vi "R3_Control-REVISED.vi"() -> ()   [LabVIEW 2016]
uses:
  R3 Reactor Status v1.ctl
  R3 PR pH Manual Control.ctl
  R3 Pump Manual Control.ctl
  R3Variables.lvlib
panel:
  in  "R3 PR pH Manual Control":T1
  out "pH and DO":T2(graph)
  in  "pH AR  Manual Control":bool
  out "AR pH Intercept":dbl
  out "AR pH slope":dbl
  in  "AR pH Calibrate":bool
  in  "Reactor 3 AR pH Manual Control":T3
  in  "AR pH Control":T4={" pH Set Point"=7.5, " pH Tolerance"=0.1, "Reaction Time (s)"=15.0, "Pump On Time (s)"=3.0}
  in  "SBR Timing":T5={"AR feeding"=0.0, "AR Decant"=0.0, "Anoxic feeding (min)"=40.0, "Anaerobic Time (min)"=53.0, "Anaerobic feeding (min)"=5.0, "Anoxic Time (min)"=60.0, "Aerobic Time (min) "=60.0, "Settle (min)"=20.0, "Decant (min)"=2.0}
  in  "R3 Pumps Manual Control":T6
  out "R3 Reactor Status":T7 {"DO (mg/L)" format="%#_3g"; "pH 1" format="%#_3g"}
  out "Elapsed Time":dbl
  out "DO Intercept":dbl
  out "DO Slope":dbl
  out "PR pH Intercept":dbl
  out "PR pH Slope":dbl
  in  "PR pH Control":T4={" pH Set Point"=7.5, " pH Tolerance"=0.1, "Reaction Time (s)"=15.0, "Pump On Time (s)"=3.0}
  in  "Pumps Manual Control":bool
  in  "pH PR Manual Control":bool
  in  "DO Calibrate":bool
  in  "PR pH Calibrate":bool
  # "On: Manual Mode\nOff: SBR Mode"
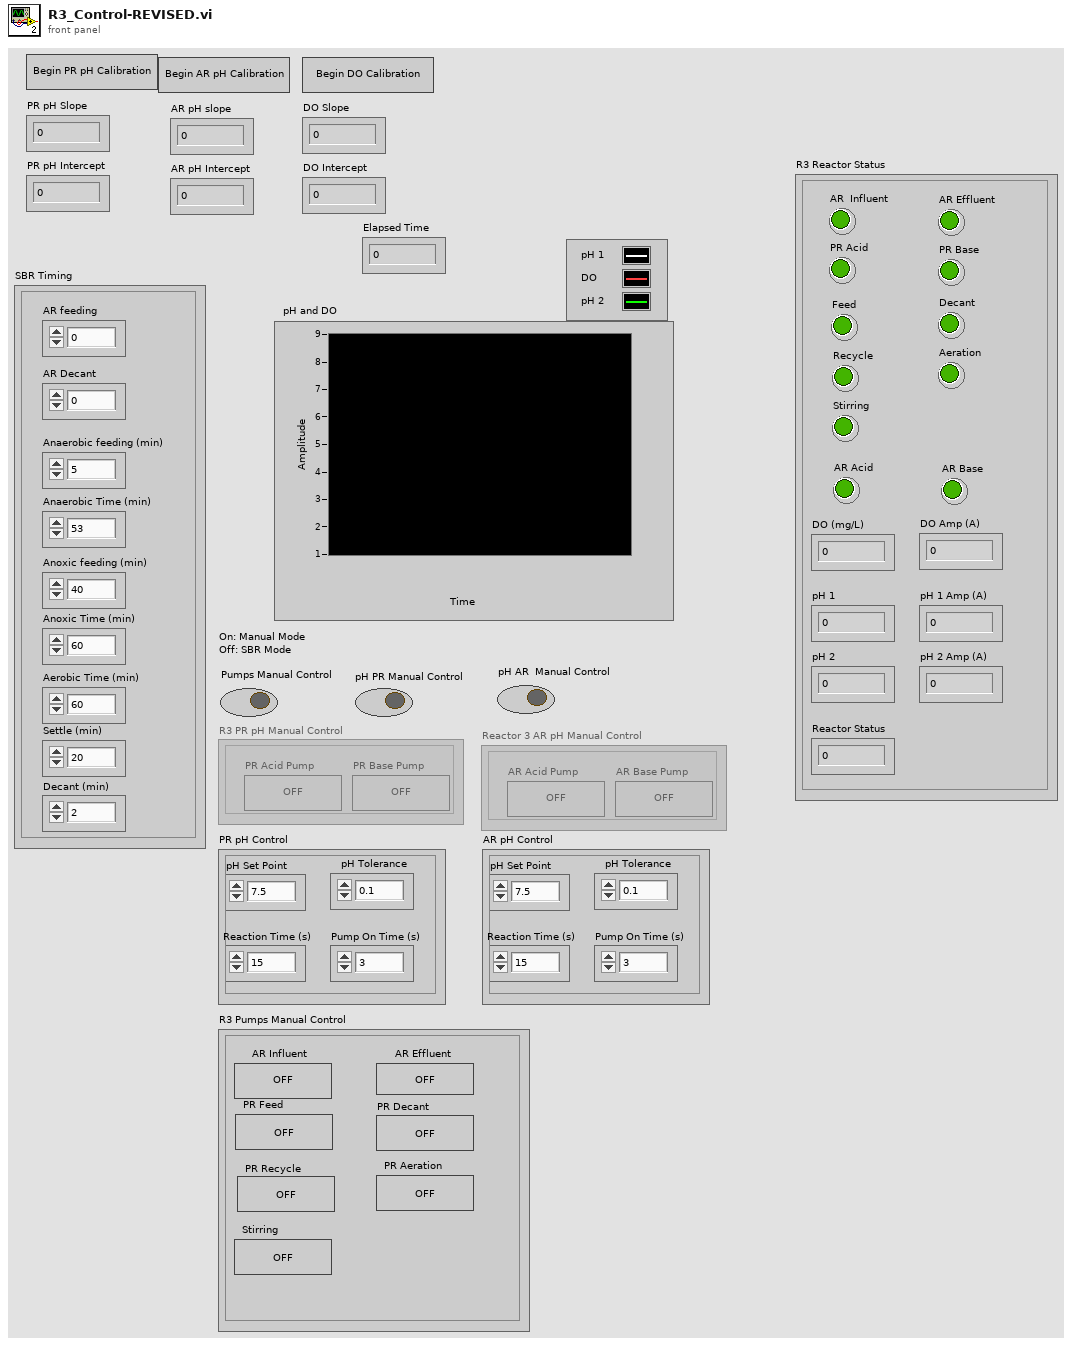
[diagram p1: front panel]
types:
  T1 = typedef "R3Variables.lvlib/R3 PR pH Manual Control.ctl" = cluster{"PR Acid Pump":bool, "PR Base Pump":bool}
  T2 = cluster{"pH 1 Amp (A)":dbl, "DO (mg/L)":dbl, "pH 2 Amp (A)":dbl}
  T3 = cluster{"AR Acid Pump":bool, "AR Base Pump":bool}
  T4 = cluster{" pH Set Point":dbl, " pH Tolerance":dbl, "Reaction Time (s)":dbl, "Pump On Time (s)":dbl}
  T5 = cluster{"AR feeding":dbl, "AR Decant":dbl, "Anoxic feeding (min)":dbl, "Anaerobic Time (min)":dbl, "Anaerobic feeding (min)":dbl, "Anoxic Time (min)":dbl, "Aerobic Time (min) ":dbl, "Settle (min)":dbl, "Decant (min)":dbl}
  T6 = cluster{"AR Influent":bool, "AR Effluent":bool, "PR Feed":bool, "PR Decant":bool, "PR Recycle":bool, "PR Aeration":bool, "Stirring":bool}
  T7 = typedef "R3Variables.lvlib/R3 Reactor Status v1.ctl" = cluster{"AR  Influent":bool, "AR Effluent":bool, "PR Acid":bool, "PR Base":bool, "Feed":bool, "Aeration":bool, "Decant":bool, "pH 1":dbl, "DO (mg/L)":dbl, "pH 1 Amp (A)":dbl, "DO Amp (A)":dbl, "Recycle":bool, "Stirring":bool, "Reactor Status":dbl, "AR Acid":bool, "AR Base":bool, "pH 2":dbl, "pH 2 Amp (A)":dbl}
  T8 = cluster{"pH 1 Amp (A)":dbl, "DO (mg/L)":dbl, "pH 2 Amp (A)":dbl}[]
  T9 = enum8{"Enabled", "Disabled", "Disabled and Grayed Out"}
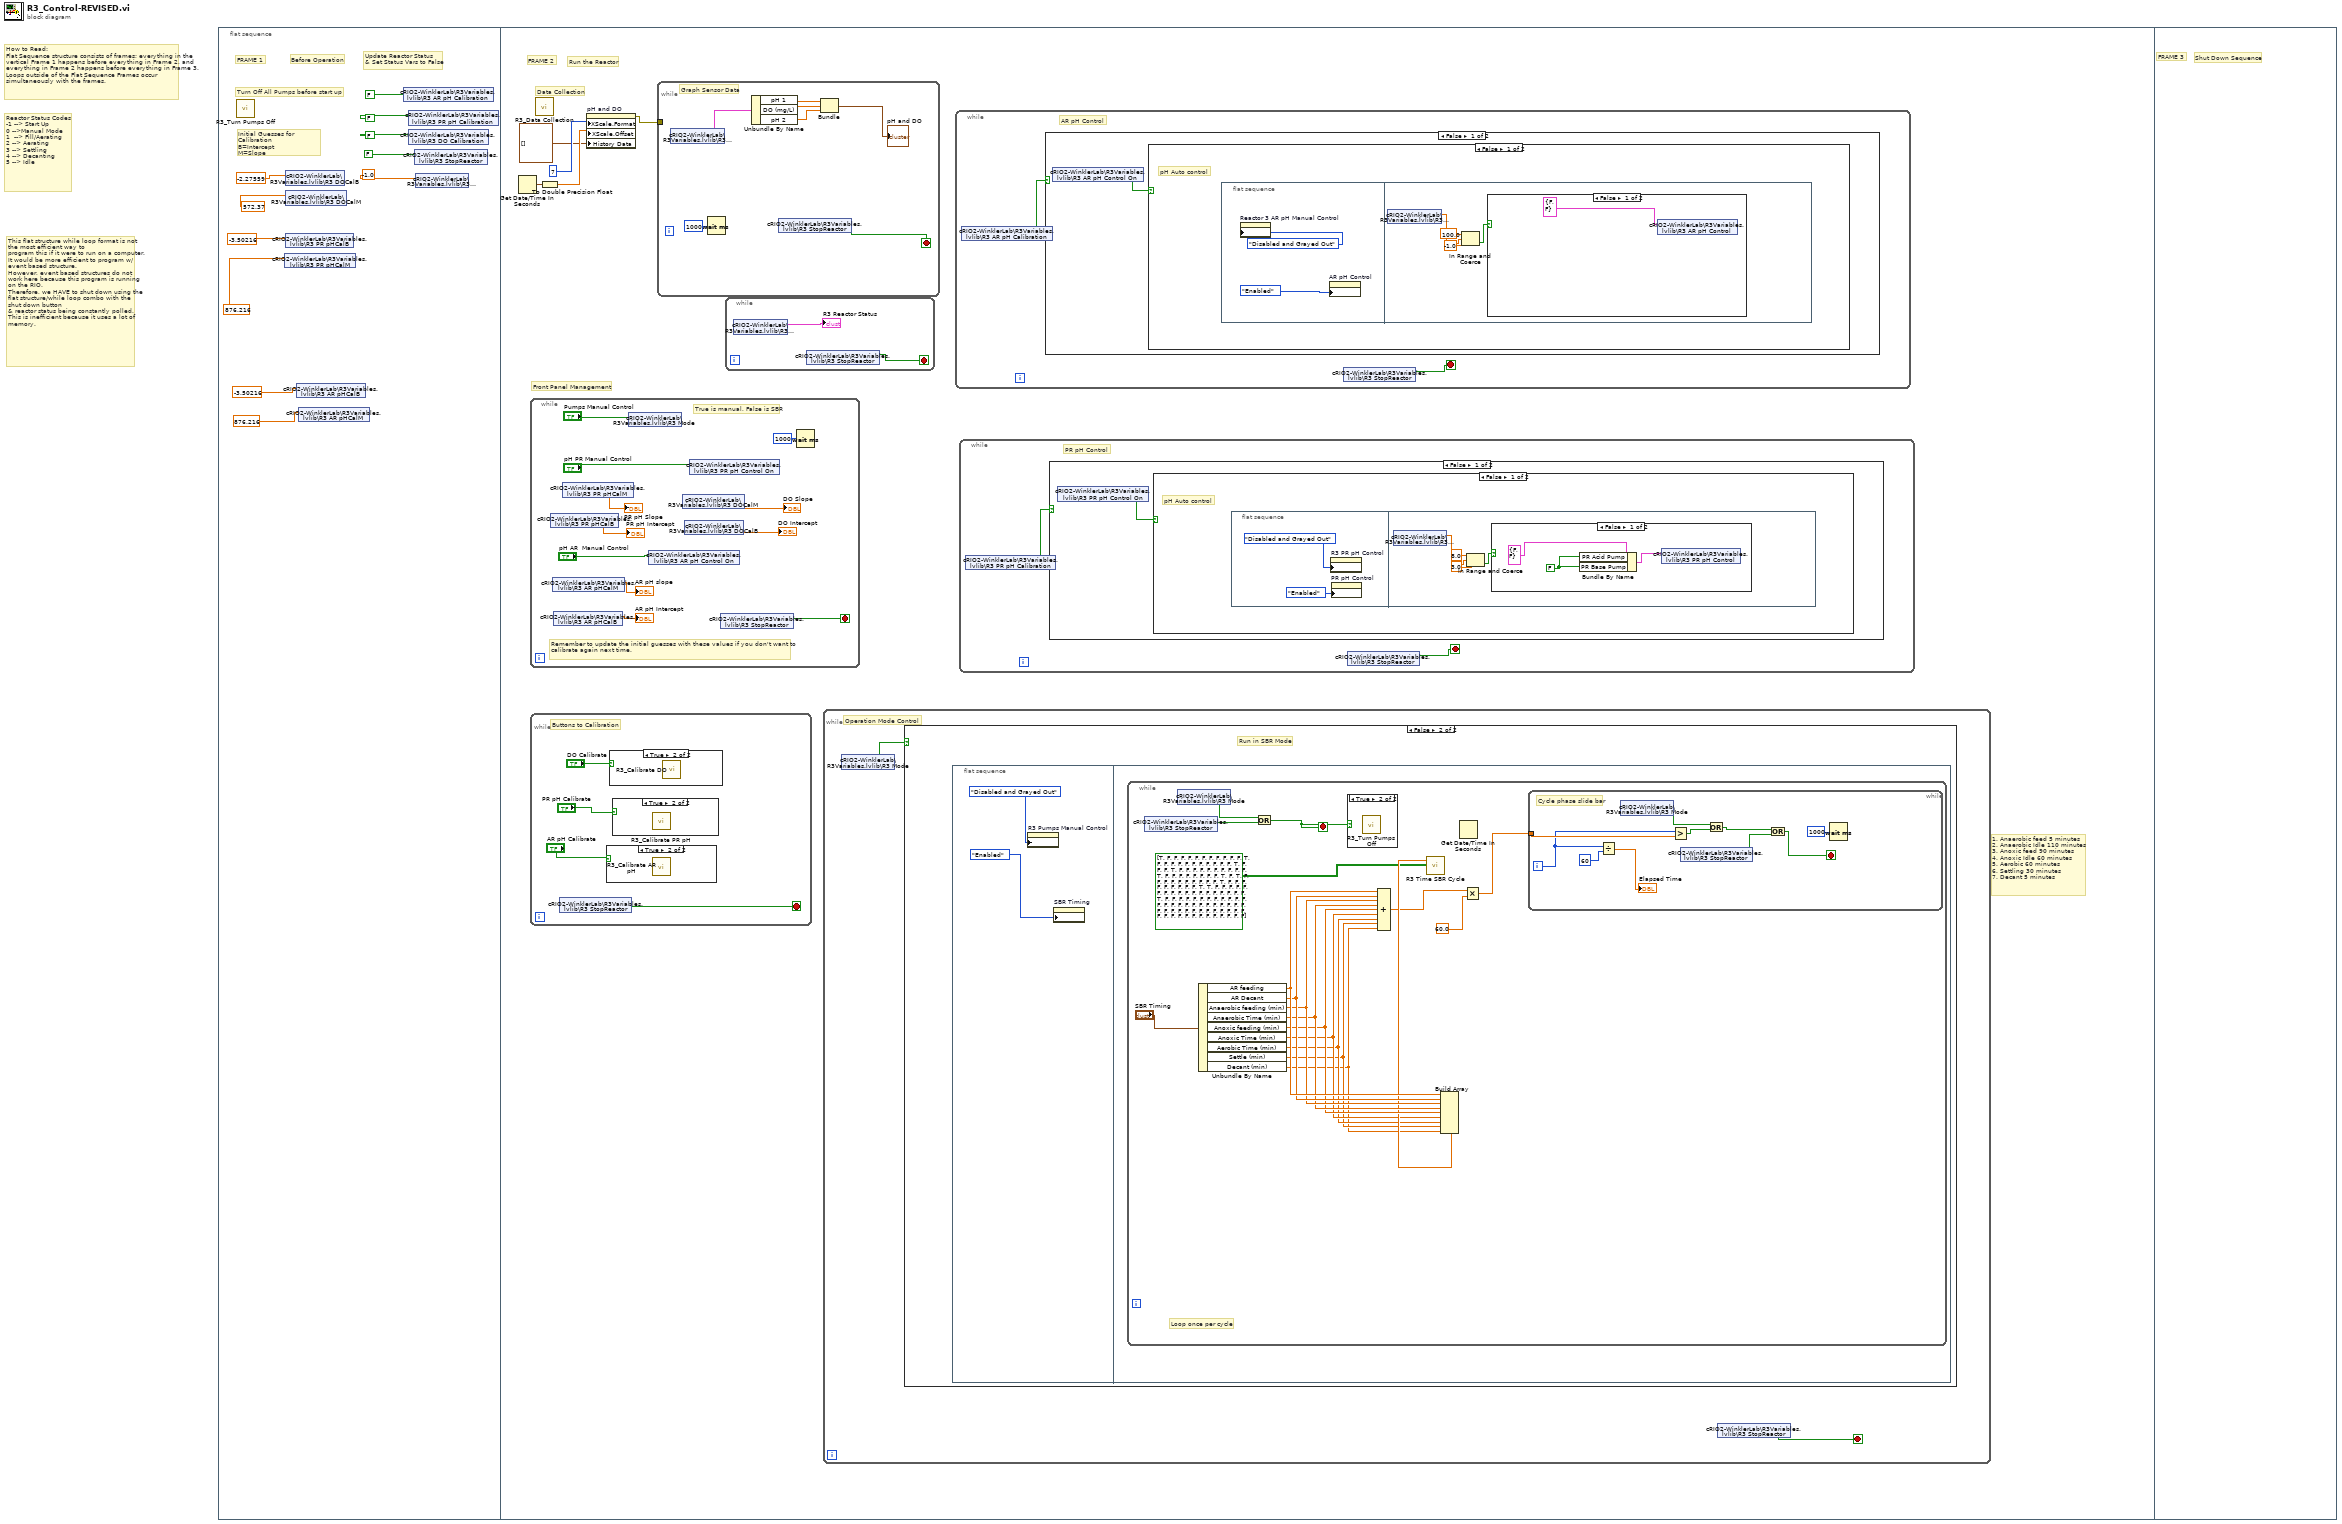
[diagram p0: block diagram]
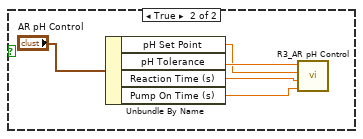
[diagram p2: hidden frame]
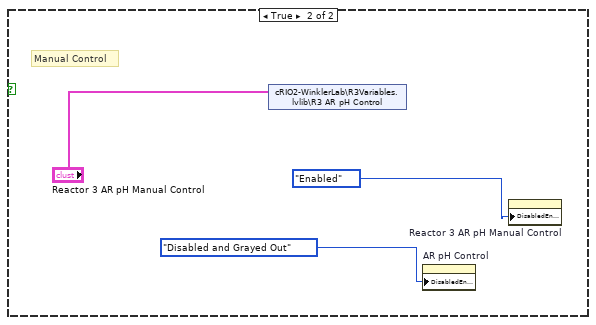
[diagram p3: hidden frame]
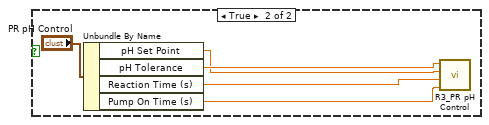
[diagram p8: hidden frame]
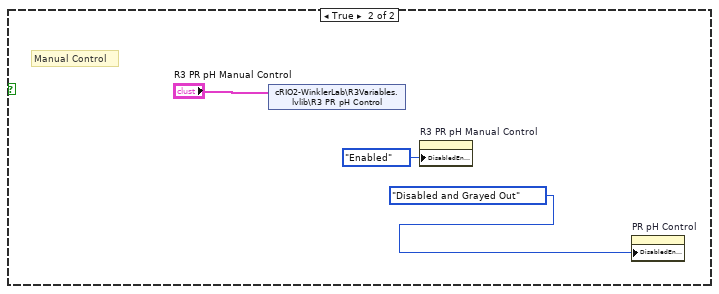
[diagram p9: hidden frame]
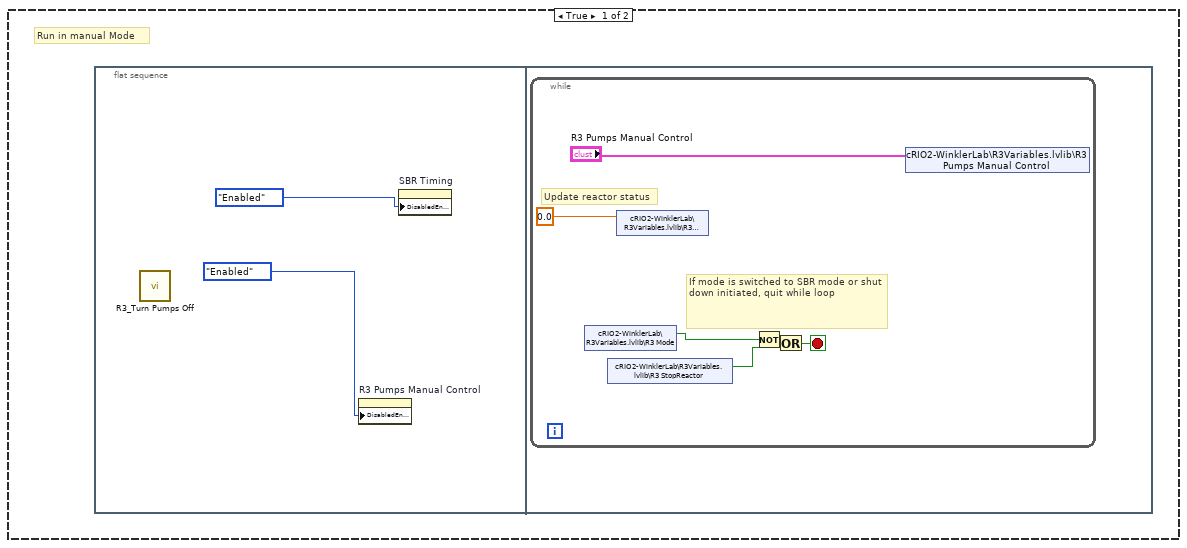
[diagram p11: hidden frame]
diagram:
  # "Reactor Status Codes\n-1 --> Start Up\n0 -->Manual Mode\n1  --> Fill/Aerating\n2 --> Aerating\n3 --> Settling\n4 --> Decanting\n5 --> Idle"
  # "How to Read:\nFlat Sequence structure consists of frames; everything in the vertical Frame 1 happens before everything in Frame 2, and everything in Frame 2 happens before everything in Frame 3.\nLoops outside of the Flat Sequence Frames occur simultaneously with the frames."
  # "This flat structure while loop format is not the most efficient way to \nprogram this if it were to run on a computer.\nIt would be more efficient to program w/ event based structure.\nHowever, event based structures do not work here because this program is running on the RIO.\nTherefore, we HAVE to shut down using the flat structure/while loop combo with the shut down button \n& reactor status being constantly polled.\nThis is inefficient because it uses a lot of memory."
  n1 = flat-sequence {
    frame #0 {
      # "Initial Guesses for Calibration\nB=Intercept\nM=Slope"
      # "Update Reactor Status \n& Set Status Vars to False"
      # "Turn Off All Pumps before start up"
      # "FRAME 1"
      # "Before Operation"
      n2 = call "R3_Turn Pumps Off.vi"() -> ()  [unwired: 12 in]
      n3 = shared-variable "cRIO2-WinklerLab\\R3Variables.lvlib\\R3 PR pHCalM"(876.216 ("R1pHCalM")) -> ()  [unwired: 1 in, 1 out]
      n4 = shared-variable "cRIO2-WinklerLab\\R3Variables.lvlib\\R3 DOCalB"(-2.27559 ("R1DOxCalB")) -> ()  [unwired: 1 in, 1 out]
      n5 = shared-variable "cRIO2-WinklerLab\\R3Variables.lvlib\\R3 DOCalM"(572.37 ("R1DOxCalM")) -> ()  [unwired: 1 in, 1 out]
      n6 = shared-variable "cRIO2-WinklerLab\\R3Variables.lvlib\\R3 PR pHCalB"(-3.50216 ("R1pHCalB")) -> ()  [unwired: 1 in, 1 out]
      n7 = shared-variable "cRIO2-WinklerLab\\R3Variables.lvlib\\R3 AR pHCalB"(-3.50216 ("pH Amperage")) -> ()  [unwired: 1 in, 1 out]
      n8 = shared-variable "cRIO2-WinklerLab\\R3Variables.lvlib\\R3 AR pHCalM"(876.216 ("Buffer Solution pH")) -> ()  [unwired: 1 in, 1 out]
      n9 = shared-variable "cRIO2-WinklerLab\\R3Variables.lvlib\\R3 AR pH Calibration"(FALSE ("Begin Calibration")) -> ()  [unwired: 1 in, 1 out]
      n10 = shared-variable "cRIO2-WinklerLab\\R3Variables.lvlib\\R3 PR pH Calibration"(FALSE ("pH Calibration")) -> ()  [unwired: 1 in, 1 out]
      n11 = shared-variable "cRIO2-WinklerLab\\R3Variables.lvlib\\R3 DO Calibration"(FALSE ("DO Calibration")) -> ()  [unwired: 1 in, 1 out]
      n12 = shared-variable "cRIO2-WinklerLab\\R3Variables.lvlib\\R3 StopReactor"(FALSE ("R1Stop Reactor")) -> ()  [unwired: 1 in, 1 out]
      n13 = shared-variable "cRIO2-WinklerLab\\R3Variables.lvlib\\R3 Phase"(-1.0) -> ()  [unwired: 1 in, 1 out]
    }
    frame #1 {
      # "1. Anaerobic feed 5 minutes\n2. Anaerobic Idle 110 minutes \n3. Anoxic feed 90 minutes\n4. Anoxic Idle 60 minutes\n5. Aerobic 60 minutes\n6. Settling 30 minutes\n7. Decant 5 minutes"
      # "Front Panel Management"
      # "Data Collection"
      # "FRAME 2"
      # "Run the Reactor"
      n14 = Get Date/Time In Seconds() -> (seconds since 1Jan1904=w16:timestamp)
      n15 = while {
        stop <- w75 stop-if-true
        # "Remember to update the initial guesses with these values if you don't want to calibrate again next time."
        # "True is manual, False is SBR"
        n16 = shared-variable "cRIO2-WinklerLab\\R3Variables.lvlib\\R3 PR pHCalB"() -> (→"PR pH Intercept":dbl)  [unwired: 1 in, 1 out]
        n17 = shared-variable "cRIO2-WinklerLab\\R3Variables.lvlib\\R3 AR pHCalM"() -> (→"AR pH slope":dbl)  [unwired: 1 in, 1 out]
        n18 = shared-variable "cRIO2-WinklerLab\\R3Variables.lvlib\\R3 AR pHCalB"() -> (→"AR pH Intercept":dbl)  [unwired: 1 in, 1 out]
        n19 = shared-variable "cRIO2-WinklerLab\\R3Variables.lvlib\\R3 PR pHCalM"() -> (→"PR pH Slope":dbl)  [unwired: 1 in, 1 out]
        n20 = shared-variable "cRIO2-WinklerLab\\R3Variables.lvlib\\R3 Mode"("Pumps Manual Control") -> ()  [unwired: 1 in, 1 out]
        n21 = shared-variable "cRIO2-WinklerLab\\R3Variables.lvlib\\R3 AR pH Control On"("pH AR  Manual Control") -> ()  [unwired: 1 in, 1 out]
        n22 = shared-variable "cRIO2-WinklerLab\\R3Variables.lvlib\\R3 DOCalM"() -> (→"DO Slope":dbl)  [unwired: 1 in, 1 out]
        n23 = shared-variable "cRIO2-WinklerLab\\R3Variables.lvlib\\R3 DOCalB"() -> (→"DO Intercept":dbl)  [unwired: 1 in, 1 out]
        n24 = shared-variable "cRIO2-WinklerLab\\R3Variables.lvlib\\R3 PR pH Control On"("pH PR Manual Control") -> ()  [unwired: 1 in, 1 out]
        n25 = shared-variable "cRIO2-WinklerLab\\R3Variables.lvlib\\R3 StopReactor"() -> (w75:bool)  [unwired: 1 in, 1 out]
        n26 = Wait (ms)(milliseconds to wait=u32 1000) -> ()  [unwired: 1 out]
      }
      n27 = while {
        stop <- w45 stop-if-true
        # "Buttons to Calibration"
        n28 = shared-variable "cRIO2-WinklerLab\\R3Variables.lvlib\\R3 StopReactor"() -> (w45:bool)  [unwired: 1 in, 1 out]
        n29 = case shown="True" "AR pH Calibrate" {
          frame False {
          }
          frame True {
            n30 = call "R3_Calibrate AR pH.vi"() -> ()  [unwired: 12 in]
          }
        }
        n31 = case shown="True" "DO Calibrate" {
          frame False {
          }
          frame True {
            n32 = call "R3_Calibrate DO.vi"() -> ()  [unwired: 12 in]
          }
        }
        n33 = case shown="True" "PR pH Calibrate" {
          frame False {
          }
          frame True {
            n34 = call "R3_Calibrate PR pH.vi"() -> ()  [unwired: 12 in]
          }
        }
      }
      n35 = call "R3_Data Collection.vi"() -> ()  [unwired: 12 in]
      n36 = To Double Precision Float(number=w16) -> (double precision float=w14:dbl)
      n37 = property on="pH and DO" class="WFChart (strict)"("XScale.Format"=u8 7 ("X Scale.Display Format:Format"), "XScale.Offset"=w14, "History Data"=T8 []) -> (error out=w13:errorcluster)  [unwired: 2 in, 1 out]
      n38 = while {
        tunnel: w13 -> [_]
        stop <- w41 stop-if-true
        # "Graph Sensor Data"
        n39 = shared-variable "cRIO2-WinklerLab\\R3Variables.lvlib\\R3 Status"() -> (w39:T7)  [unwired: 1 in, 1 out]
        n40 = Wait (ms)(milliseconds to wait=u32 1000) -> ()  [unwired: 1 out]
        n41 = Unbundle By Name(w39) -> ("pH 1"=w42:dbl, "DO (mg/L)"=w43:dbl, "pH 2"=w37:dbl)
        n42 = shared-variable "cRIO2-WinklerLab\\R3Variables.lvlib\\R3 StopReactor"() -> (w41:bool)  [unwired: 1 in, 1 out]
        n43 = Bundle("pH 1"=w42, "DO (mg/L)"=w43, "pH 2"=w37) -> (→"pH and DO":cluster{"pH 1":dbl, "DO (mg/L)":dbl, "pH 2":dbl})  [unwired: 1 in]
      }
      n44 = while {
        stop <- w36 stop-if-true
        n45 = shared-variable "cRIO2-WinklerLab\\R3Variables.lvlib\\R3 Status"() -> (→"R3 Reactor Status":T7)  [unwired: 1 in, 1 out]
        n46 = shared-variable "cRIO2-WinklerLab\\R3Variables.lvlib\\R3 StopReactor"() -> (w36:bool)  [unwired: 1 in, 1 out]
      }
      n47 = while {
        stop <- w80 stop-if-true
        # "Operation Mode Control"
        n48 = shared-variable "cRIO2-WinklerLab\\R3Variables.lvlib\\R3 Mode"() -> (w79:bool)  [unwired: 1 in, 1 out]
        n49 = case shown="False" w79 {
          frame True {
            # "Run in manual Mode"
            n50 = flat-sequence {
              frame #0 {
                n51 = call "R3_Turn Pumps Off.vi"() -> ()  [unwired: 12 in]
                n52 = property on="R3 Pumps Manual Control" class="Clust (strict)"("DisabledEnum"=T9."Enabled" ("Disabled")) -> ()  [unwired: 2 in, 2 out]
                n53 = property on="SBR Timing" class="Clust (strict)"("DisabledEnum"=T9."Enabled" ("Disabled")) -> ()  [unwired: 2 in, 2 out]
              }
              frame #1 {
                n54 = while {
                  stop <- w87 stop-if-true
                  # "If mode is switched to SBR mode or shut \ndown initiated, quit while loop"
                  # "Update reactor status"
                  n55 = shared-variable "cRIO2-WinklerLab\\R3Variables.lvlib\\R3 Mode"() -> (w85:bool)  [unwired: 1 in, 1 out]
                  n56 = shared-variable "cRIO2-WinklerLab\\R3Variables.lvlib\\R3 StopReactor"() -> (w84:bool)  [unwired: 1 in, 1 out]
                  n57 = shared-variable "cRIO2-WinklerLab\\R3Variables.lvlib\\R3 Phase"(0.0 ("Reactor Status")) -> ()  [unwired: 1 in, 1 out]
                  n58 = Not(x=w85) -> (.not. x?=w88:bool)
                  n59 = Or(x=w88, y=w84) -> (x .or. y?=w87:bool)
                  n60 = shared-variable "cRIO2-WinklerLab\\R3Variables.lvlib\\R3 Pumps Manual Control"("R3 Pumps Manual Control") -> ()  [unwired: 1 in, 1 out]
                }
              }
            }
          }
          frame False {
            # "Run in SBR Mode"
            n61 = flat-sequence {
              frame #0 {
                n62 = property on="R3 Pumps Manual Control" class="Clust (strict)"("DisabledEnum"=T9."Disabled and Grayed Out" ("Disabled")) -> ()  [unwired: 2 in, 2 out]
                n63 = property on="SBR Timing" class="Clust (strict)"("DisabledEnum"=T9."Enabled" ("Disabled")) -> ()  [unwired: 2 in, 2 out]
              }
              frame #1 {
                n64 = while {
                  stop <- w108 stop-if-true
                  # "Loop once per cycle"
                  n65 = shared-variable "cRIO2-WinklerLab\\R3Variables.lvlib\\R3 StopReactor"() -> (w106:bool)  [unwired: 1 in, 1 out]
                  n66 = shared-variable "cRIO2-WinklerLab\\R3Variables.lvlib\\R3 Mode"() -> (w107:bool)  [unwired: 1 in, 1 out]
                  n67 = Unbundle By Name("SBR Timing") -> ("AR feeding"=w105:dbl, "AR Decant"=w104:dbl, "Anaerobic feeding (min)"=w103:dbl, "Anaerobic Time (min)"=w102:dbl, "Anoxic feeding (min)"=w101:dbl, "Anoxic Time (min)"=w95:dbl, "Aerobic Time (min)"=w94:dbl, "Settle (min)"=w93:dbl, "Decant (min)"=w92:dbl)
                  n68 = Or(x=w107, y=w106) -> (x .or. y?=w108:bool)
                  n69 = case shown="True" w108 {
                    frame False {
                    }
                    frame True {
                      n70 = call "R3_Turn Pumps Off.vi"() -> ()  [unwired: 12 in]
                    }
                  }
                  n71 = Compound Arithmetic op=ADD(w105, w104, w103, w102, w101, w95, w94, w93, w92) -> (w96:dbl)
                  n72 = Build Array(w105, w104, w103, w102, w101, w95, w94, w93, w92) -> (w100:dbl[])
                  n73 = call "R3 Time SBR Cycle.vi"("Pump Status Array"=bool[][] [[TRUE, FALSE, FALSE, FALSE, FALSE, FALSE, FALSE, FALSE, FALSE, FALSE, FALSE], [FALSE, TRUE, FALSE, FALSE, FALSE, FALSE, FALSE, FALSE, FALSE, FALSE, FALSE], [FALSE, FALSE, TRUE, FALSE, FALSE, FALSE, TRUE, FALSE, FALSE, FALSE, FALSE], [FALSE, FALSE, FALSE, FALSE, FALSE, FALSE, TRUE, FALSE, FALSE, FALSE, FALSE], [FALSE, FALSE, FALSE, FALSE, TRUE, FALSE, TRUE, FALSE, FALSE, FALSE, FALSE], [FALSE, FALSE, FALSE, FALSE, FALSE, FALSE, TRUE, FALSE, FALSE, FALSE, FALSE], [FALSE, FALSE, FALSE, FALSE, FALSE, TRUE, TRUE, FALSE, FALSE, FALSE, FALSE], [FALSE, FALSE, FALSE, FALSE, FALSE, FALSE, FALSE, FALSE, FALSE, FALSE, FALSE], [FALSE, FALSE, FALSE, TRUE, FALSE, FALSE, FALSE, FALSE, FALSE, FALSE, FALSE], [FALSE, FALSE, FALSE, FALSE, FALSE, FALSE, FALSE, FALSE, FALSE, FALSE, FALSE], [FALSE, FALSE, FALSE, FALSE, FALSE, FALSE, FALSE, FALSE, FALSE, FALSE, FALSE], [FALSE, FALSE, FALSE, FALSE, FALSE, FALSE, FALSE, FALSE, FALSE, FALSE, FALSE], [FALSE, FALSE, FALSE, FALSE, FALSE, FALSE, FALSE, FALSE, FALSE, FALSE, FALSE]], "Timing Array"=w100) -> ()  [unwired: 10 in]
                  n74 = Get Date/Time In Seconds() -> ()  [unwired: 1 out]
                  n75 = Multiply(x=w96, y=60.0) -> (x*y=w97:dbl)
                  n76 = while {
                    tunnel: w97 -> [w117]
                    i -> [w111]
                    stop <- w112 stop-if-true
                    # "Cycle phase slide bar"
                    n77 = Divide(x=w111, y=60) -> (x/y=→"Elapsed Time":dbl)
                    n78 = shared-variable "cRIO2-WinklerLab\\R3Variables.lvlib\\R3 Mode"() -> (w114:bool)  [unwired: 1 in, 1 out]
                    n79 = Greater?(x=w111, y=w117) -> (0:w115:bool)
                    n80 = shared-variable "cRIO2-WinklerLab\\R3Variables.lvlib\\R3 StopReactor"() -> (w109:bool)  [unwired: 1 in, 1 out]
                    n81 = Or(x=w114, y=w115) -> (x .or. y?=w113:bool)
                    n82 = Or(x=w113, y=w109) -> (x .or. y?=w112:bool)
                    n83 = Wait (ms)(milliseconds to wait=u32 1000) -> ()  [unwired: 1 out]
                  }
                }
              }
            }
          }
        }
        n84 = shared-variable "cRIO2-WinklerLab\\R3Variables.lvlib\\R3 StopReactor"() -> (w80:bool)  [unwired: 1 in, 1 out]
      }
      n85 = while {
        stop <- w17 stop-if-true
        # "AR pH Control"
        n86 = shared-variable "cRIO2-WinklerLab\\R3Variables.lvlib\\R3 AR pH Calibration"() -> (w18:bool)  [unwired: 1 in, 1 out]
        n87 = case shown="False" w18 {
          frame False {
            n88 = shared-variable "cRIO2-WinklerLab\\R3Variables.lvlib\\R3 AR pH Control On"() -> (w19:bool)  [unwired: 1 in, 1 out]
            n89 = case shown="False" w19 {
              frame False {
                # "pH Auto control"
                n90 = flat-sequence {
                  frame #0 {
                    n91 = property on="Reactor 3 AR pH Manual Control" class="Clust (strict)"("DisabledEnum"=T9."Disabled and Grayed Out" ("Disabled")) -> ()  [unwired: 2 in, 2 out]
                    n92 = property on="AR pH Control" class="Clust (strict)"("DisabledEnum"=T9."Enabled" ("Disabled")) -> ()  [unwired: 2 in, 2 out]
                  }
                  frame #1 {
                    n93 = shared-variable "cRIO2-WinklerLab\\R3Variables.lvlib\\R3 Phase"() -> (w24:dbl)  [unwired: 1 in, 1 out]
                    n94 = In Range and Coerce(upper limit=100.0, x=w24, lower limit=-1.0) -> (In Range?=w22:bool)  [unwired: 1 out]
                    n95 = case shown="False" w22 {
                      frame False {
                        n96 = shared-variable "cRIO2-WinklerLab\\R3Variables.lvlib\\R3 AR pH Control"(T3 {"AR Acid Pump"=FALSE, "AR Base Pump"=FALSE} ("R3 AR pH Control")) -> ()  [unwired: 1 in, 1 out]
                      }
                      frame True {
                        n97 = Unbundle By Name("AR pH Control") -> ("pH Set Point"=w27:dbl, "pH Tolerance"=w28:dbl, "Reaction Time (s)"=w30:dbl, "Pump On Time (s)"=w29:dbl)
                        n98 = call "R3_AR pH Control.vi"("Pump On Time (s)"=w29, "Reaction Time (s)"=w30, "pH Set Point"=w27, "pH Tolerance"=w28) -> ()  [unwired: 8 in]
                      }
                    }
                  }
                }
              }
              frame True {
                # "Manual Control"
                n99 = shared-variable "cRIO2-WinklerLab\\R3Variables.lvlib\\R3 AR pH Control"("Reactor 3 AR pH Manual Control") -> ()  [unwired: 1 in, 1 out]
                n100 = property on="AR pH Control" class="Clust (strict)"("DisabledEnum"=T9."Disabled and Grayed Out" ("Disabled")) -> ()  [unwired: 2 in, 2 out]
                n101 = property on="Reactor 3 AR pH Manual Control" class="Clust (strict)"("DisabledEnum"=T9."Enabled" ("Disabled")) -> ()  [unwired: 2 in, 2 out]
              }
            }
          }
          frame True {
          }
        }
        n102 = shared-variable "cRIO2-WinklerLab\\R3Variables.lvlib\\R3 StopReactor"() -> (w17:bool)  [unwired: 1 in, 1 out]
      }
      n103 = while {
        stop <- w48 stop-if-true
        # "PR pH Control"
        n104 = shared-variable "cRIO2-WinklerLab\\R3Variables.lvlib\\R3 PR pH Calibration"() -> (w49:bool)  [unwired: 1 in, 1 out]
        n105 = case shown="False" w49 {
          frame False {
            n106 = shared-variable "cRIO2-WinklerLab\\R3Variables.lvlib\\R3 PR pH Control On"() -> (w50:bool)  [unwired: 1 in, 1 out]
            n107 = case shown="False" w50 {
              frame False {
                # "pH Auto control"
                n108 = flat-sequence {
                  frame #0 {
                    n109 = property on="R3 PR pH Control" class="Clust (strict)"("DisabledEnum"=T9."Disabled and Grayed Out" ("Disabled")) -> ()  [unwired: 2 in, 2 out]
                    n110 = property on="PR pH Control" class="Clust (strict)"("DisabledEnum"=T9."Enabled" ("Disabled")) -> ()  [unwired: 2 in, 2 out]
                  }
                  frame #1 {
                    n111 = shared-variable "cRIO2-WinklerLab\\R3Variables.lvlib\\R3 Phase"() -> (w55:dbl)  [unwired: 1 in, 1 out]
                    n112 = In Range and Coerce(upper limit=8.0, x=w55, lower limit=3.0) -> (In Range?=w53:bool)  [unwired: 1 out]
                    n113 = case shown="False" w53 {
                      frame False {
                        w59 = FALSE
                        n114 = Bundle By Name(cluster=T1 {"PR Acid Pump"=FALSE, "PR Base Pump"=FALSE} ("R3 PR pH Control"), "PR Acid Pump"=w59, "PR Base Pump"=w59) -> (w57:T1)
                        n115 = shared-variable "cRIO2-WinklerLab\\R3Variables.lvlib\\R3 PR pH Control"(w57) -> ()  [unwired: 1 in, 1 out]
                      }
                      frame True {
                        n116 = Unbundle By Name("PR pH Control") -> ("pH Set Point"=w60:dbl, "pH Tolerance"=w61:dbl, "Reaction Time (s)"=w63:dbl, "Pump On Time (s)"=w62:dbl)
                        n117 = call "R3_PR pH Control.vi"("Pump On Time (s)"=w62, "Reaction Time (s)"=w63, "pH Set Point"=w60, "pH Tolerance"=w61) -> ()  [unwired: 8 in]
                      }
                    }
                  }
                }
              }
              frame True {
                # "Manual Control"
                n118 = shared-variable "cRIO2-WinklerLab\\R3Variables.lvlib\\R3 PR pH Control"("R3 PR pH Manual Control") -> ()  [unwired: 1 in, 1 out]
                n119 = property on="R3 PR pH Manual Control" class="Clust (strict)"("DisabledEnum"=T9."Enabled" ("Disabled")) -> ()  [unwired: 2 in, 2 out]
                n120 = property on="PR pH Control" class="Clust (strict)"("DisabledEnum"=T9."Disabled and Grayed Out" ("Disabled")) -> ()  [unwired: 2 in, 2 out]
              }
            }
          }
          frame True {
          }
        }
        n121 = shared-variable "cRIO2-WinklerLab\\R3Variables.lvlib\\R3 StopReactor"() -> (w48:bool)  [unwired: 1 in, 1 out]
      }
    }
    frame #2 {
      # "FRAME 3"
      # "Shut Down Sequence"
    }
  }
